vi "Process Primary.vi"(11 "Arilou in":refnum<class "Arilou.lvclass">) -> (2 "New Elements":refnum<class "Element.lvclass">[](array[class]), 3 "Arilou out":refnum<class "Arilou.lvclass">)   [LabVIEW 2021, in "Arilou.lvclass"]
uses:
  Arilou.lvclass
  Element/Element.lvclass
  Weapons/Laser/Laser.lvclass
  Re-use Libraries/Vector 2D/Vector 2D.lvclass
  Ship/Ship.lvclass
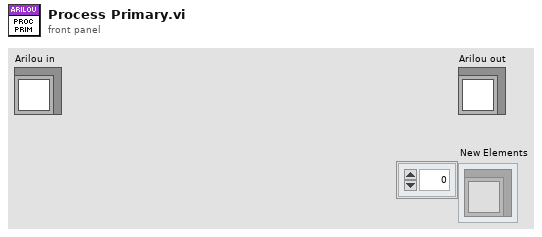
[diagram p1: front panel]
types:
  T1 = typedef "Element.lvclass/Player Type.ctl" = enum16{"Neutral", "Player 1", "Player 2"}
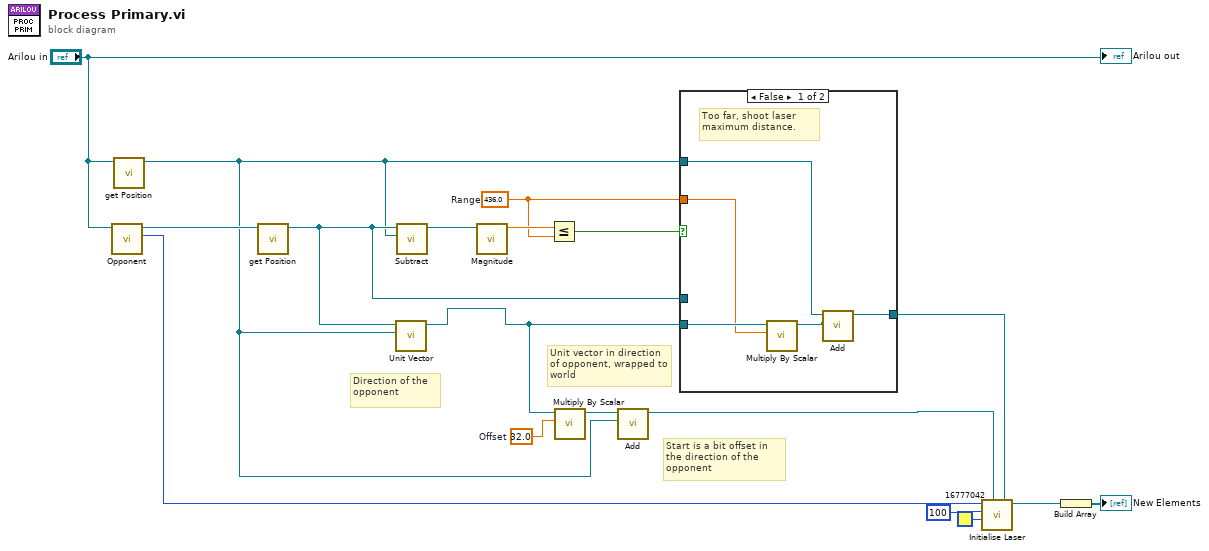
[diagram p0: block diagram]
diagram:
  w6 = sgl 436.0  # Range
  w7 = sgl 32.0  # Offset
  # "Unit vector in direction of opponent, wrapped to world"
  # "Start is a bit offset in the direction of the opponent"
  # "Direction of the opponent"
  n1 = call "Opponent.vi"("Element in"="Arilou in") -> ("Player Type"=w13:T1, "Opponent out"=w14:refnum<class "Element.lvclass">)  [unwired: 9 in]
  n2 = call "get Position.vi"("Element in"="Arilou in") -> ("Position"=w4:refnum<class "Vector 2D.lvclass">)  [unwired: 10 in]
  n3 = call "get Position.vi"("Element in"=w14) -> ("Position"=w5:refnum<class "Vector 2D.lvclass">)  [unwired: 10 in]
  n4 = call "Unit Vector.vi"("Position 2"=w4, "Position 1"=w5) -> ("Unit Vector In Direction"=w3:refnum<class "Vector 2D.lvclass">)  [unwired: 9 in]
  n5 = call "Subtract.vi"("B"=w4, "A"=w5) -> ("A-B"=w9:refnum<class "Vector 2D.lvclass">)  [unwired: 9 in]
  n6 = call "Magnitude.vi"("A"=w9) -> ("Magnitude"=w12:sgl)  [unwired: 10 in]
  n7 = Less Or Equal?(x=w12, y=w6) -> (x <= y?=w11:bool)
  n8 = call "Multiply By Scalar.vi"("x"=w7, "A"=w3) -> ("Ax"=w8:refnum<class "Vector 2D.lvclass">)  [unwired: 9 in]
  n9 = call "Add.vi"("B"=w4, "A"=w8) -> ("A+B"=w1:refnum<class "Vector 2D.lvclass">)  [unwired: 9 in]
  n10 = case shown="False" w11 {
    tunnel: w5 -> [_ w24]
    tunnel: w4 -> [w21 _]
    tunnel: w3 -> [w22 _]
    tunnel: [w23 w24] -> w2
    tunnel: w6 -> [w19 _]
    frame False {
      # "Too far, shoot laser maximum distance."
      n11 = call "Multiply By Scalar.vi"("x"=w19, "A"=w22) -> ("Ax"=w20:refnum<class "Vector 2D.lvclass">)  [unwired: 9 in]
      n12 = call "Add.vi"("B"=w20, "A"=w21) -> ("A+B"=w23:refnum<class "Vector 2D.lvclass">)  [unwired: 9 in]
    }
    frame True {
      # "Ships is in distance. Start a bit offset , just end directly at the target"
    }
  }
  n13 = call "Initialise Laser.vi"("Endpoint"=w2, "Origin"=w1, "Colour"=u32 16777042, "Damage"=100, "Player Type"=w13) -> ("Laser out"=w17:refnum<class "Laser.lvclass">)  [unwired: 6 in]
  n14 = Build Array(w17) -> (→"New Elements":refnum<class "Laser.lvclass">[])
  "Arilou out" <- "Arilou in"
